vi "updateTimer.vi"(8 "error in (no error)":errorcluster, 11 "deviceHeartbeat in":refnum<class "deviceHeartbeat.lvclass">) -> (0 "error out":errorcluster, 2 "getStatus?":bool, 3 "deviceHeartbeat out":refnum<class "deviceHeartbeat.lvclass">)   [LabVIEW 2016, in "deviceHeartbeat.lvclass"]
uses:
  deviceHeartbeat.lvclass
  deviceHeartbeat.lvclass/deviceHeartbeat.ctl
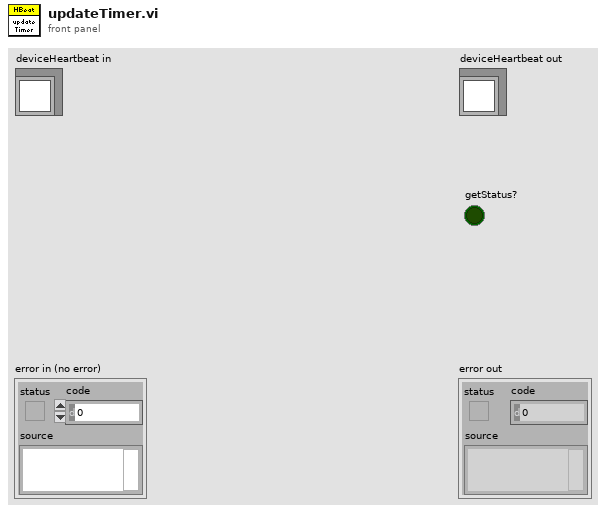
[diagram p1: front panel]
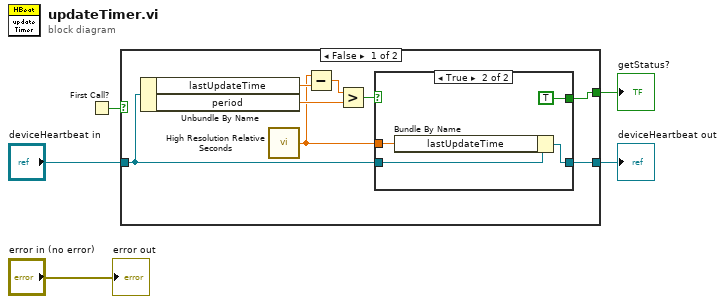
[diagram p0: block diagram]
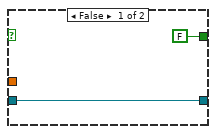
[diagram p2: hidden frame]
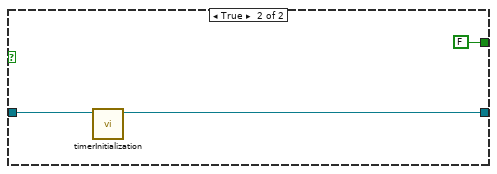
[diagram p3: hidden frame]
diagram:
  n1 = First Call?() -> (First Call?: T/F=w2:bool)
  n2 = case shown="False" w2 {
    tunnel: [w8 FALSE ("getStatus?")] -> w4
    tunnel: "deviceHeartbeat in" -> [w7 w22]
    tunnel: [w6 w21] -> w1
    frame False {
      n3 = Unbundle By Name(w7) -> ("lastUpdateTime"=w13:dbl, "period"=w11:dbl)
      n4 = call <vilib>:"High Resolution Relative Seconds.vi"() -> ("relative seconds"=w9:dbl)
      n5 = Subtract(x=w9, y=w13) -> (x-y=w12:dbl)
      n6 = Greater?(x=w12, y=w11) -> (0:w10:bool)
      n7 = case shown="True" w10 {
        tunnel: w7 -> [w15 w18]
        tunnel: [w15 w16] -> w6
        tunnel: [FALSE ("getStatus?") TRUE ("getStatus?")] -> w8
        tunnel: w9 -> [_ w17]
        frame False {
        }
        frame True {
          n8 = Bundle By Name(cluster=w18, "lastUpdateTime"=w17) -> (w16:refnum<class "deviceHeartbeat.lvclass">)
        }
      }
    }
    frame True {
      n9 = call "timerInitialization.vi"("deviceHeartbeat in"=w22) -> ("deviceHeartbeat out"=w21:refnum<class "deviceHeartbeat.lvclass">)  [unwired: 9 in, 1 out]
    }
  }
  "deviceHeartbeat out" <- w1
  "getStatus?" <- w4
  "error out" <- "error in (no error)"
